vi "Power Supply Status Cluster to Map.vi"(8 "error in (no error)":errorcluster, 10 "Power Supply Status":T1) -> (0 "error out":errorcluster, 2 "Power Supply Status Map":map{string, dbl}(c390))   [LabVIEW 2024, in "Power Supply.lvlib"]
uses:
  Power Supply.lvlib
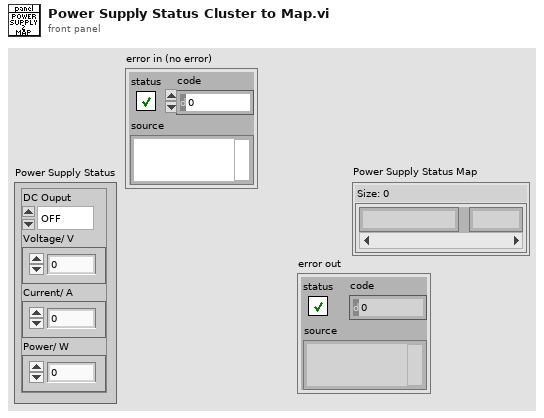
[diagram p1: front panel]
types:
  T1 = cluster{"DC Ouput":enum16{"OFF", "ON"}, "Voltage/ V":dbl, "Current/ A":dbl, "Power/ W":dbl}
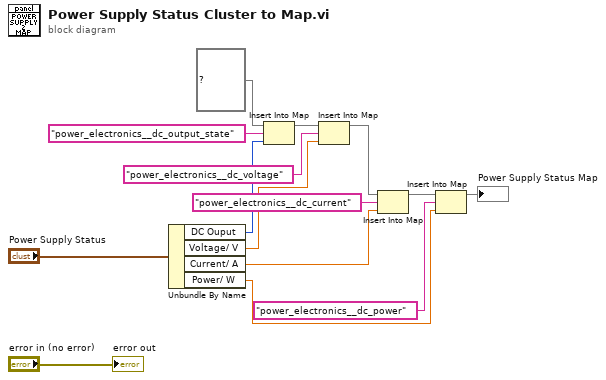
[diagram p0: block diagram]
diagram:
  n1 = Unbundle By Name("Power Supply Status") -> ("DC Ouput"=w9:enum16{"OFF", "ON"}, "Voltage/ V"=w7:dbl, "Current/ A"=w3:dbl, "Power/ W"=w2:dbl)
  n2 = Insert Into Map(map in=map{string, dbl} {} ("Power Supply Status Map"), key="power_electronics__dc_output_state", value=w9) -> (map out=w13:map{string, dbl})  [unwired: 2 out]
  n3 = Insert Into Map(map in=w13, key="power_electronics__dc_voltage", value=w7) -> (map out=w12:map{string, dbl})  [unwired: 2 out]
  n4 = Insert Into Map(map in=w12, key="power_electronics__dc_current", value=w3) -> (map out=w11:map{string, dbl})  [unwired: 2 out]
  n5 = Insert Into Map(map in=w11, key="power_electronics__dc_power", value=w2) -> (map out=→"Power Supply Status Map":map{string, dbl})  [unwired: 2 out]
  "error out" <- "error in (no error)"
